vi "Vision Processing.vi"(4 "error in (no error)":errorcluster, 6 "CameraDevRef":T1) -> ()   [LabVIEW 2011]
uses:
  <vilib>/Rock Robotics/WPI/Camera/WPI_CameraDevRef.ctl
  Robot Global Data.vi
  <vilib>/vision/NI_Vision_Development_Module.lvlib
panel:
  in  "Run Calculations":bool
  in  "Manual Overide":bool
  out "Turret Rotation":dbl
  out "Target X Coord":dbl
  out "Target Distance":dbl
  out "Target Y Coord":dbl
  out "Distance Array":dbl[](array[numeric])
  in  "Scaler":dbl=0.85
  in  "Lower Speed Limit":dbl=0.05
  out "Number of Rectangles Visible":dbl
  out "Y Position Array":dbl[](array[numeric])
  out "X Position Array":dbl[](array[numeric])
  in  "View":bool
  out "Target Info":T2(array[cluster])
  in  "Area Size Limit":i32=444
  in  "Particle Count Limit":i32=8
  in  "Score Limits":T3={"Rect Coverage"=76.0, "Aspect Ratio"=40.0, "X Edge Strength"=40.0, "Y Edge Strength"=60.0}
  in  "Processing":enum32{"Color", "Intensity", "Intensity Open"}(tab)=enum."Intensity Open"
  in  "Luminance":i32=255
  in  "Saturation":i32=255
  in  "Hue":i32(knob)=65 scale=0.0..255.0
  in  "Margins":cluster{"Hue":i32, "Sat":i32, "Lum":i32}={"Hue"=20, "Sat"=27, "Lum"=30} {"Sat" scale=0.0..40.0; "Lum" scale=0.0..40.0; "Hue" scale=0.0..40.0}
  in  "Range":cluster{"Lower value":sgl, "Upper value":sgl}={"Lower value"=150.0, "Upper value"=255.0} {"Lower value" scale=0.0..255.0; "Upper value" scale=0.0..255.0}
  in  "Range":cluster{"Lower value":sgl, "Upper value":sgl}={"Lower value"=123.804344, "Upper value"=255.0} {"Lower value" scale=0.0..255.0; "Upper value" scale=0.0..255.0}
  in  "View":bool
  out "Processed Image":T4(plugin-control)
  out "Original Image":T4(plugin-control)
  # "Instructions:\nProcessing the reflective tape that is illuminated by a ring light can be based\non color or light intensity.\nParticles within the image are scored by rectangle coverage, aspect ratio, and\nfor being hollow with a bold edge. A particle is considered a target if all scores\nare above the score limits. Particles can be annotated -- surrounded by\na rectangle and scores drawn to the left .\nTo control the number of particles being scored, use the count limit and the size\nlimit."
  # "To debug, Enable using the View button.\nFor color processing, you can click in the image to select the color for processing."
  # "Enable by clicking the View button.\nGreen scores are above the limit, orange are below. Inner/outer rect\nindicates all passed."
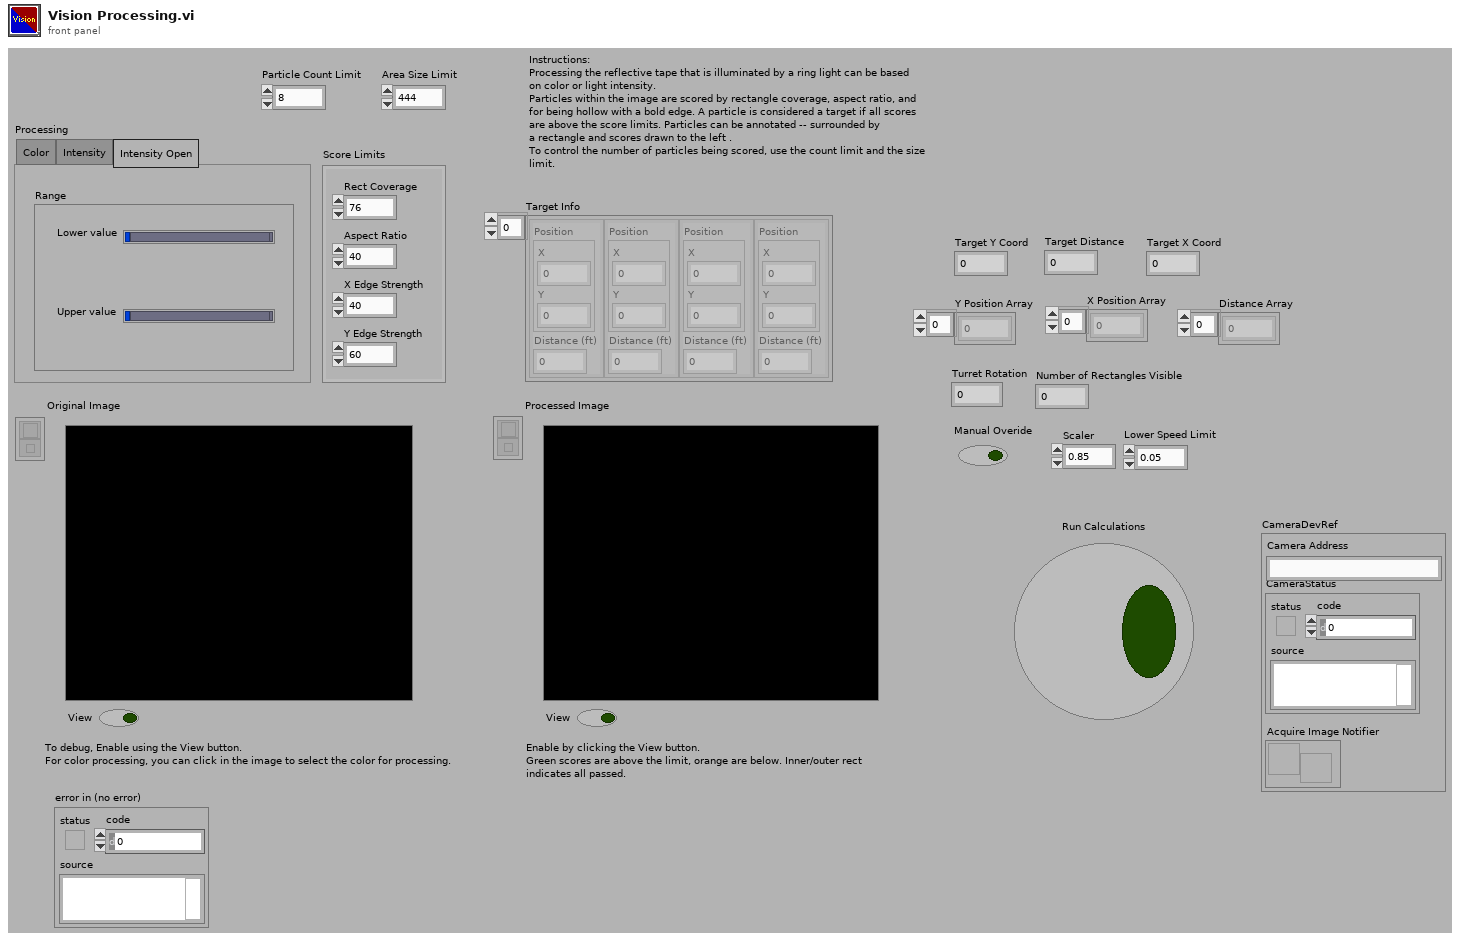
[diagram p1: front panel]
types:
  T1 = typedef "WPI_CameraDevRef.ctl" = cluster{"Camera Address":string, "CameraStatus":errorcluster, "Acquire Image Notifier":refnum<notifier>}
  T2 = cluster{"Position":cluster{"X":dbl, "Y":dbl}, "Distance (ft)":dbl}[]
  T3 = cluster{"Rect Coverage":dbl, "Aspect Ratio":dbl, "X Edge Strength":dbl, "Y Edge Strength":dbl}
  T4 = typedef "IMAQ Image.ctl" = refnum<image>
  T5 = typedef "Image Type" = u32
  T6 = enum32{"AutoM", "Close", "Dilate", "Erode", "Gradient", "Gradient out", "Gradient in", "Hit miss", "Open", "PClose", "POpen", "Thick", "Thin"}
  T7 = typedef "WPI_CameraImageSize.ctl" = enum16{"640x480", "320x240", "160x120"}
  T8 = cluster{"fps":i32, "compression":i32, "Image Size":T7}
  T9 = cluster{cluster{"Left":dbl, "Top":dbl, "Right":dbl, "Bottom":dbl}, dbl[]}[]
  T10 = cluster{"Left":dbl, "Top":dbl, "Right":dbl, "Bottom":dbl}
  T11 = cluster{"Target Center (-1 to 1)":cluster{"X":dbl, "Y":dbl}, "Distance (ft)":dbl}
  T12 = cluster{"Target Center (-1 to 1)":cluster{"X":dbl, "Y":dbl}, "Distance (ft)":dbl}[]
  T13 = cluster{"Axis 1":dbl, "Axis 2":dbl, "Axis 3":dbl, "Axis 4":dbl, "Axis 5":dbl, "Axis 6":dbl, "Button 1":bool, "Button 2":bool, "Button 3":bool, "Button 4":bool, "Button 5":bool, "Button 6":bool, "Button 7":bool, "Button 8":bool, "Button 9":bool, "Button 10":bool, "Button 11":bool, "Button 12":bool}
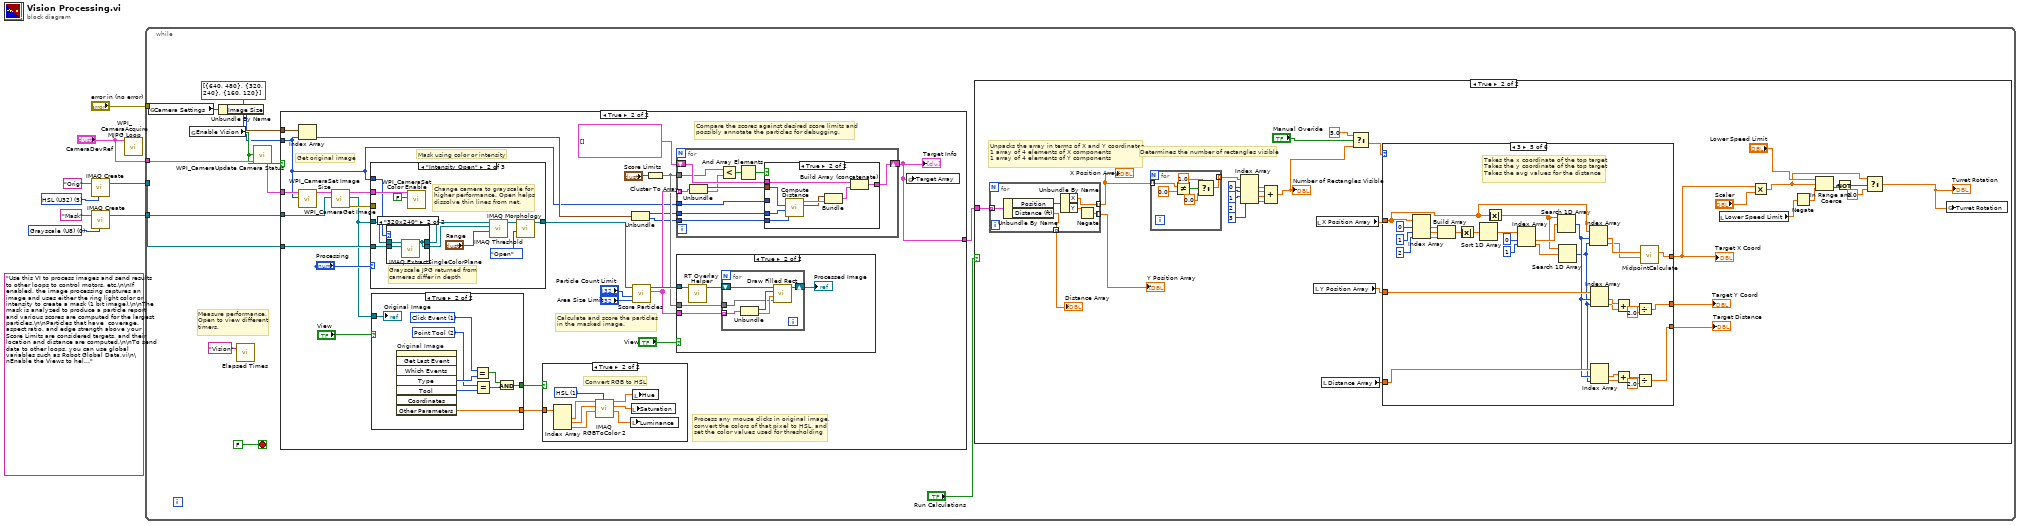
[diagram p0: block diagram]
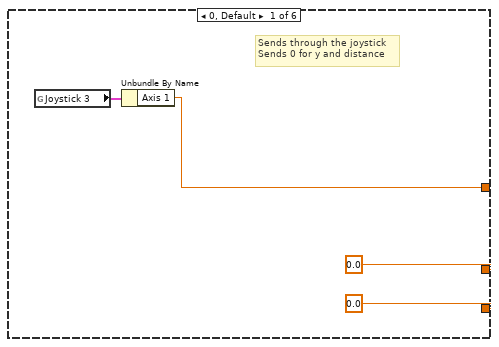
[diagram p3: hidden frame]
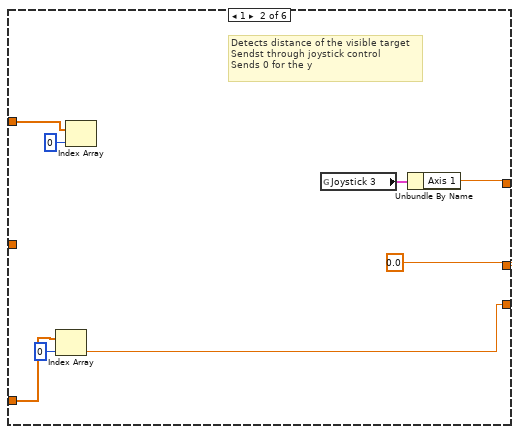
[diagram p4: hidden frame]
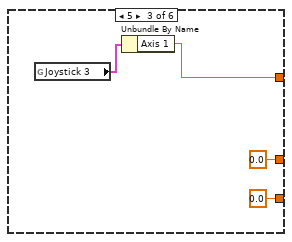
[diagram p5: hidden frame]
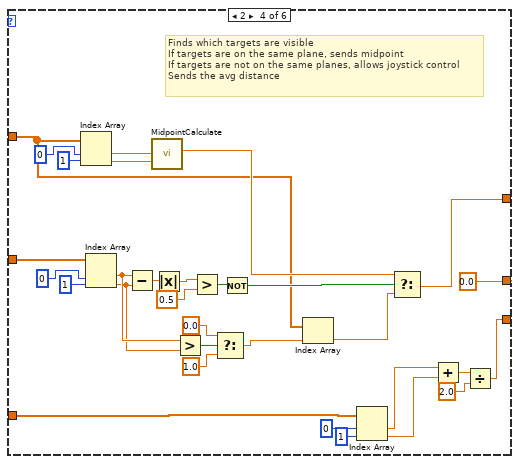
[diagram p6: hidden frame]
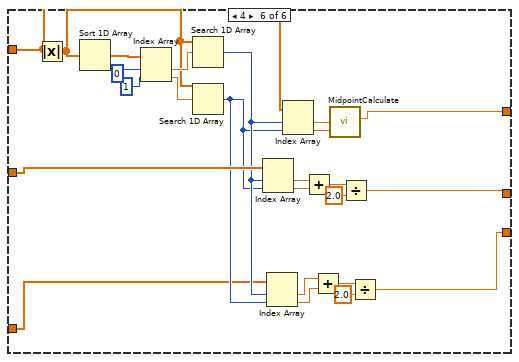
[diagram p7: hidden frame]
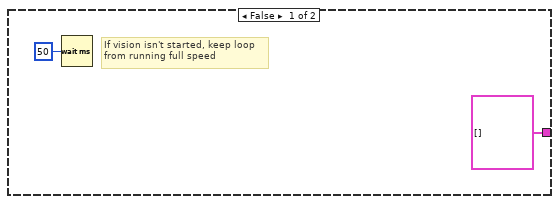
[diagram p8: hidden frame]
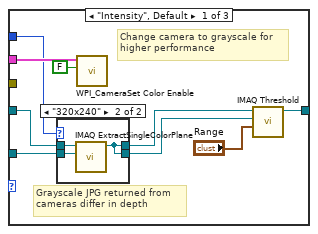
[diagram p10: hidden frame]
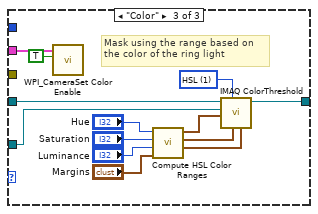
[diagram p13: hidden frame]
diagram:
  w3 = T5 0 items=["Grayscale (U8)", "Grayscale (I16)", "Grayscale (SGL)", "Complex (CSG)", "RGB (U32)", "HSL (U32)", "RGB (U64)", "Grayscale (U16)"] ("Image Type")
  (unwired) "Use this VI to process images and send results to other loops to control motors, etc.\n\nIf enabled, the image processing captures an image and uses either the ring light color or intensity to create a mask (1 bit image).\n\nThe mask is analyzed to produce a particle report and various scores are computed for the largest particles.\n\nParticles that have  coverage, aspect ratio, and edge strength above your Score Limits are considered targets, and their location and distance are computed.\n\nTo send data to other loops, you can use global variables such as Robot Global Data.vi\n\nEnable the Views to help debug color settings. Disable the View to speed up processing."
  w7 = T5 5 items=["Grayscale (U8)", "Grayscale (I16)", "Grayscale (SGL)", "Complex (CSG)", "RGB (U32)", "HSL (U32)", "RGB (U64)", "Grayscale (U16)"] ("Image Type")
  n1 = call "IMAQ Create"("Image Name"="Orig", "Image Type"=w7) -> ("New Image"=w6:T4)  [unwired: 2 in, 2 out]
  n2 = call "IMAQ Create"("Image Name"="Mask", "Image Type"=w3) -> ("New Image"=w1:T4)  [unwired: 2 in, 2 out]
  n3 = call <vilib>:"WPI_CameraAcquire MJPG Loop.vi"("CameraDevRef"="CameraDevRef") -> ()  [unwired: 11 in]
  n4 = while {
    tunnel: w6 -> [w19]
    tunnel: "CameraDevRef" -> [w18]
    tunnel: "error in (no error)" -> [_]
    tunnel: w1 -> [w14]
    stop <- FALSE stop-if-true
    # "Measure performance.\nOpen to view different\ntimers."
    n5 = global read "Robot Global Data.vi" "Camera Settings"() -> (w12:T8)
    n6 = global read "Robot Global Data.vi" "Enable Vision"() -> (w16:bool)
    n7 = Unbundle By Name(w12) -> ("Image Size"=w11:T7)
    n8 = call "Elapsed Times.vi"("Call Name"="Vision") -> ()  [unwired: 2 in, 1 out]
    n9 = call <vilib>:"WPI_CameraUpdate Camera Status.vi"("CameraDevRef In"=w18, "Enable Vision"=w16) -> ("CameraDevRef Out"=w17:T1)  [unwired: 3 in]
    n10 = case shown="True" w16 {
      tunnel: w19 -> [_ w186]
      tunnel: w17 -> [_ w182]
      tunnel: w14 -> [_ w173]
      tunnel: cluster{i32, i32}[] [{640, 480}, {320, 240}, {160, 120}] -> [_ w177]
      tunnel: w11 -> [_ w170]
      tunnel: [T2 [] w171] -> w10
      frame False {
        # "If vision isn't started, keep loop\nfrom running full speed"
        n11 = Wait (ms)(milliseconds to wait=u32 50) -> ()  [unwired: 1 out]
      }
      frame True {
        # "Compare the scores against desired score limits and\npossibly annotate the particles for debugging."
        # "Process any mouse clicks in original image,\nconvert the colors of that pixel to HSL, and\nset the color values used for thresholding"
        # "Calculate and score the particles\nin the masked image."
        # "Mask using color or intensity"
        # "Get original image"
        n12 = call <vilib>:"WPI_CameraSet Image Size.vi"("Image Size"=w170, "CameraDevRef"=w182) -> ("CameraDevRef Out"=w183:T1)  [unwired: 8 in, 1 out]
        n13 = Index Array(array=w177, index=w170) -> (element=w174:cluster{i32, i32})
        n14 = call <vilib>:"WPI_CameraGet Image.vi"("Image"=w186, "CameraDevRef"=w183) -> ("error out"=w184:errorcluster, "Image Out"=w172:T4, "CameraDevRef Out"=w185:T1)  [unwired: 7 in]
        n15 = case shown="\"Intensity Open\"" "Processing" {
          tunnel: w172 -> [w208 w220 w246]
          tunnel: [w211 w225 w245] -> w180
          tunnel: w185 -> [w209 w223 w236]
          tunnel: w184 -> [_ _ _]
          tunnel: w173 -> [w207 w221 w234]
          tunnel: w170 -> [w206 w222 _]
          frame "Intensity", Default {
            # "Grayscale JPG returned from\ncameras differ in depth"
            # "Change camera to grayscale for\nhigher performance"
            n16 = case shown="\"320x240\"" w206 {
              tunnel: w208 -> [w214 w217]
              tunnel: w207 -> [w213 w216]
              tunnel: [w214 w215] -> w205
              tunnel: [w213 w215] -> w204
              frame "640x480", Default {
              }
              frame "320x240" {
                n17 = call "IMAQ ExtractSingleColorPlane"("Image Dst"=w216, "Image Src"=w217) -> ("Image Dst Out"=w215:T4)  [unwired: 8 in, 1 out]
              }
            }
            n18 = call <vilib>:"WPI_CameraSet Color Enable.vi"("Color Enabled"=FALSE, "CameraDevRef"=w209) -> ()  [unwired: 8 in, 2 out]
            n19 = call "IMAQ Threshold"("Range"="Range", "Image Dst"=w204, "Image Src"=w205) -> ("Image Dst Out"=w211:T4)  [unwired: 3 in, 5 out]
          }
          frame "Intensity Open" {
            # "Grayscale JPG returned from\ncameras differ in depth"
            # "Change camera to grayscale for\nhigher performance. Open helps\ndissolve thin lines from net."
            n20 = case shown="\"320x240\"" w222 {
              tunnel: w220 -> [w230 w233]
              tunnel: w221 -> [w229 w232]
              tunnel: [w230 w231] -> w219
              tunnel: [w229 w231] -> w218
              frame "640x480", Default {
              }
              frame "320x240" {
                n21 = call "IMAQ ExtractSingleColorPlane"("Image Dst"=w232, "Image Src"=w233) -> ("Image Dst Out"=w231:T4)  [unwired: 8 in, 1 out]
              }
            }
            n22 = call <vilib>:"WPI_CameraSet Color Enable.vi"("Color Enabled"=FALSE, "CameraDevRef"=w223) -> ()  [unwired: 8 in, 2 out]
            n23 = call "IMAQ Threshold"("Range"="Range", "Image Dst"=w218, "Image Src"=w219) -> ("Image Dst Out"=w226:T4)  [unwired: 3 in, 5 out]
            n24 = call "IMAQ Morphology"("Operation"=T6."Open", "Image Src"=w226) -> ("Image Dst Out"=w225:T4)  [unwired: 8 in, 1 out]
          }
          frame "Color" {
            w244 = u16 1 items=["RGB", "HSL", "HSV", "HSI"] ("Color Mode")
            # "Mask using the range based on\nthe color of the ring light"
            n25 = call <vilib>:"WPI_CameraSet Color Enable.vi"("Color Enabled"=TRUE, "CameraDevRef"=w236) -> ()  [unwired: 8 in, 2 out]
            n26 = call "Compute HSL Color Ranges.vi"("Margins"="Margins", "Luminance"="Luminance", "Saturation"="Saturation", "Hue"="Hue") -> ("Lum Range"=w241:cluster{i32, i32}, "Sat Range"=w242:cluster{i32, i32}, "Hue Range"=w243:cluster{i32, i32})  [unwired: 5 in]
            n27 = call "IMAQ ColorThreshold"("Blue or Luma or Val or Inten Range"=w241, "Green or Sat Range"=w242, "Color Mode"=w244, "Red or Hue Range"=w243, "Image Dst"=w234, "Image Src"=w246) -> ("Image Dst Out"=w245:T4)  [unwired: 4 in, 1 out]
          }
        }
        n28 = case shown="True" "View" {
          tunnel: w172 -> [_ w266]
          tunnel: [_ w261] -> w179
          tunnel: [_ w258] -> w178
          frame False {
          }
          frame True {
            w259 = 2 items=["None", "Selection Tool", "Point Tool", "Line Tool", "Rectangle Tool", "Oval Tool", "Polygon Tool", "ClosedFreehandTool", "Annulus Tool", "Rotated Rectangle Tool", "Zoom Tool", "Pan Tool", "Polyline Tool", "Freehand Tool"] ("Tool")
            w260 = 1 items=["No Event"=0, "Click Event"=1, "Draw Event"=2, "Size Event"=4, "Scroll Event"=5, "Double Click Event"=8] ("Type")
            n29 = invoke on="Original Image" class="ImageControl" method="Get Last Event"() -> ("Type"=w262:i32, "Tool"=w265:i32, "Other Parameters"=w258:sgl[])  [unwired: 8 in, 5 out]
            n30 = Equal?(x=w260, y=w262) -> (x = y?=w263:bool)
            n31 = Equal?(x=w259, y=w265) -> (x = y?=w264:bool)
            n32 = And(x=w263, y=w264) -> (x .and. y?=w261:bool)
            "Original Image" <- w266
          }
        }
        n33 = case shown="True" w179 {
          tunnel: w178 -> [_ w203]
          frame False {
          }
          frame True {
            w202 = u16 1 items=["RGB", "HSL", "HSV", "HSI", "CIE L*a*b*", "CIE XYZ"] ("Color Mode")
            # "Convert RGB to HSL"
            n34 = Index Array(array=w203) -> (element #1=w201:sgl, element #2=w199:sgl, element #3=w197:sgl)  [unwired: 3 in]
            n35 = call "IMAQ RGBToColor 2"("Color Mode"=w202, "Blue value"=w197, "Green value"=w199, "Red value"=w201) -> ("Blue or Luma or Val or Inten or Z or b*value"=w196:dbl, "Green or Sat or Y or a* value"=w198:dbl, "Red or Hue or X or L* value"=w200:dbl)  [unwired: 4 in, 1 out]
            n36 = local write "Luminance"(w196) -> ()
            n37 = local write "Saturation"(w198) -> ()
            n38 = local write "Hue"(w200) -> ()
          }
        }
        n39 = Unbundle(w174) -> (w176:i32, w175:i32)
        n40 = call "Score Particles.vi"("Area Size Limit"="Area Size Limit", "Particle Count Limit"="Particle Count Limit", "Image Refnum in"=w180) -> ("Scored Particle Info"=w191:T9, "Image Refnum out"=w194:T4)  [unwired: 7 in]
        n41 = Cluster To Array(cluster="Score Limits") -> (array=w189:dbl[])
        n42 = for {
          shift-right: [w276] -> w171
          shift-left: T2 [] -> [w277]
          tunnel: w176 -> [w275]
          tunnel: w191 -> [w273] mode=indexing
          tunnel: w189 -> [w268]
          tunnel: w170 -> [w272]
          tunnel: w175 -> [w267]
          n43 = Unbundle(w273) -> (w274:T10, w269:dbl[])
          n44 = Less?(x=w268, y=w269) -> (x < y?=w271:bool[])
          n45 = And Array Elements(Boolean array=w271) -> (logical AND=w270:bool)
          n46 = case shown="True" w270 {
            tunnel: w277 -> [w278 w286]
            tunnel: [w278 w285] -> w276
            tunnel: w274 -> [_ w281]
            tunnel: w275 -> [_ w283]
            tunnel: w272 -> [_ _]
            tunnel: w267 -> [_ w280]
            frame False {
            }
            frame True {
              n47 = call "Compute Distance.vi"("Y Image Resolution"=w280, "X Image Resolution"=w283, "Bounding Box"=w281) -> ("Target Center (-1 to 1)"=w279:cluster{"X":dbl, "Y":dbl}, "Distance (ft)"=w282:dbl)  [unwired: 7 in]
              n48 = Bundle("Target Center (-1 to 1)"=w279, "Distance (ft)"=w282) -> (w284:T11)  [unwired: 1 in]
              n49 = Build Array (concatenate)(w286, w284) -> (w285:T12)
            }
          }
        }
        "Target Info" <- w171
        n50 = case shown="True" "View" {
          tunnel: w194 -> [_ w248]
          tunnel: w191 -> [_ w250]
          tunnel: w189 -> [_ w249]
          frame False {
          }
          frame True {
            n51 = call "RT Overlay Helper.vi"("Refnum in"=w248) -> ("Refnum out"=w251:T4)  [unwired: 10 in]
            n52 = for {
              shift-right: [w256] -> w247
              shift-left: w251 -> [w257]
              tunnel: w250 -> [w253] mode=indexing
              tunnel: w249 -> [w252]
              n53 = Unbundle(w253) -> (w254:T10, w255:dbl[])
              n54 = call "Draw Filled Rect.vi"("Limits"=w252, "Scores"=w255, "Bounding Box"=w254, "image in"=w257) -> ("image out"=w256:T4)  [unwired: 7 in]
            }
            "Processed Image" <- w247
          }
        }
        n55 = global write "Robot Global Data.vi" "Target Array"(w171) -> ()
      }
    }
    n56 = case shown="True" "Run Calculations" {
      tunnel: w10 -> [_ w22]
      frame False {
      }
      frame True {
        # "Determines the number of rectangles visible"
        # "Unpacks the array in terms of X and Y coordinates\n1 array of 4 elements of X components\n1 array of 4 elements of Y components"
        n57 = for {
          tunnel: [w165] -> w23 mode=indexing
          tunnel: [w166] -> w33 mode=indexing
          tunnel: w22 -> [w163] mode=indexing
          tunnel: [w162] -> w42 mode=indexing
          n58 = Unbundle By Name(w163) -> ("Position"=w167:cluster{"X":dbl, "Y":dbl}, "Distance (ft)"=w162:dbl)
          n59 = Unbundle By Name(w167) -> ("X"=w166:dbl, "Y"=w164:dbl)
          n60 = Negate(x=w164) -> (-x=w165:dbl)
        }
        "X Position Array" <- w33
        "Y Position Array" <- w23
        "Distance Array" <- w42
        n61 = for {
          tunnel: w33 -> [w57] mode=indexing
          tunnel: [w53] -> w32 mode=indexing
          n62 = Not Equal?(x=w57, y=0.0) -> (x != y?=w56:bool)
          n63 = Select(t=1.0, s=w56, f=0.0) -> (s? t:f=w53:dbl)
        }
        n64 = Index Array(array=w32, index #1=0 ("index"), index #2=1 ("index"), index #3=2 ("index"), index #4=3 ("index")) -> (element #1=w30:dbl, element #2=w31:dbl, element #3=w29:dbl, element #4=w28:dbl)
        n65 = Compound Arithmetic op=ADD(w30, w31, w29, w28) -> (w21:dbl)
        "Number of Rectangles Visible" <- w21
        n66 = local read "Y Position Array"() -> (w46:dbl[])
        n67 = local read "X Position Array"() -> (w34:dbl[])
        n68 = local read "Distance Array"() -> (w47:dbl[])
        n69 = Select(t=5.0, s="Manual Overide", f=w21) -> (s? t:f=w50:dbl)
        n70 = case shown="3" w50 {
          tunnel: w34 -> [_ w65 _ w76 w123 w156]
          tunnel: [w61 w63 w73 w94 w120 w153] -> w45
          tunnel: [0.0 ("X") 0.0 ("X") 0.0 ("X") 0.0 ("X") w111 w147] -> w43
          tunnel: [0.0 ("X") w68 0.0 ("X") w87 w106 w139] -> w44
          tunnel: w46 -> [_ _ _ w103 w119 w152]
          tunnel: w47 -> [_ w70 _ w86 w118 w144]
          frame 0, Default {
            # "Sends through the joystick\nSends 0 for y and distance"
            n71 = global read "Robot Global Data.vi" "Joystick 3"() -> (w62:T13)
            n72 = Unbundle By Name(w62) -> ("Axis 1"=w61:dbl)
          }
          frame 1 {
            # "Detects distance of the visible target\nSendst through joystick control\nSends 0 for the y"
            n73 = Index Array(array=w70, index=0) -> (element=w68:dbl)
            n74 = Index Array(array=w65, index=0) -> ()  [unwired: 1 out]
            n75 = global read "Robot Global Data.vi" "Joystick 3"() -> (w64:T13)
            n76 = Unbundle By Name(w64) -> ("Axis 1"=w63:dbl)
          }
          frame 5 {
            n77 = global read "Robot Global Data.vi" "Joystick 3"() -> (w74:T13)
            n78 = Unbundle By Name(w74) -> ("Axis 1"=w73:dbl)
          }
          frame 2 {
            # "Finds which targets are visible\nIf targets are on the same plane, sends midpoint\nIf targets are not on the same planes, allows joystick control\nSends the avg distance"
            n79 = Index Array(array=w76, index #1=0 ("index"), index #2=1 ("index")) -> (element #1=w92:dbl, element #2=w91:dbl)
            n80 = Index Array(array=w103, index #1=0 ("index"), index #2=1 ("index")) -> (element #1=w82:dbl, element #2=w81:dbl)
            n81 = Subtract(x=w82, y=w81) -> (x-y=w100:dbl)
            n82 = call "MidpointCalculate.vi"("X2"=w91, "X1"=w92) -> ("Midpoint"=w95:dbl)  [unwired: 9 in]
            n83 = Absolute Value(x=w100) -> (abs(x)=w99:dbl)
            n84 = Greater?(x=w82, y=w81) -> (0:w80:bool)
            n85 = Greater?(x=w99, y=0.5) -> (0:w96:bool)
            n86 = Select(t=0.0, s=w80, f=1.0) -> (s? t:f=w77:dbl)
            n87 = Not(x=w96) -> (.not. x?=w97:bool)
            n88 = Index Array(array=w76, index=w77) -> (element=w75:dbl)
            n89 = Index Array(array=w86, index #1=0 ("index"), index #2=1 ("index")) -> (element #1=w85:dbl, element #2=w84:dbl)
            n90 = Select(t=w95, s=w97, f=w75) -> (s? t:f=w94:dbl)
            n91 = Add(x=w85, y=w84) -> (x+y=w90:dbl)
            n92 = Divide(x=w90, y=2.0) -> (x/y=w87:dbl)
          }
          frame 3 {
            # "Takes the x coordinate of the top target\nTakes the y coordinate of the top target\nTakes the avg values for the distance"
            n93 = Index Array(array=w123, index #1=0 ("index"), index #2=1 ("index"), index #3=2 ("index")) -> (element #1=w134:dbl, element #2=w133:dbl, element #3=w132:dbl)
            n94 = Build Array(w134, w133, w132) -> (w131:dbl[])
            n95 = Absolute Value(x=w131) -> (abs(x)=w130:dbl[])
            n96 = Sort 1D Array(array=w130) -> (sorted array=w129:dbl[])
            n97 = Absolute Value(x=w123) -> (abs(x)=w124:dbl[])
            n98 = Index Array(array=w129, index #1=0 ("index"), index #2=1 ("index")) -> (element #1=w126:dbl, element #2=w125:dbl)
            n99 = Search 1D Array(1D array=w124, element=w126) -> (index of element=w117:i32)  [unwired: 1 in]
            n100 = Search 1D Array(1D array=w124, element=w125) -> (index of element=w116:i32)  [unwired: 1 in]
            n101 = Index Array(array=w123, index #1=w117, index #2=w116) -> (element #1=w122:dbl, element #2=w121:dbl)
            n102 = Index Array(array=w119, index #1=w117, index #2=w116) -> (element #1=w113:dbl, element #2=w112:dbl)
            n103 = Index Array(array=w118, index #1=w117, index #2=w116) -> (element #1=w108:dbl, element #2=w107:dbl)
            n104 = Add(x=w113, y=w112) -> (x+y=w115:dbl)
            n105 = Add(x=w108, y=w107) -> (x+y=w110:dbl)
            n106 = Divide(x=w115, y=2.0) -> (x/y=w111:dbl)
            n107 = Divide(x=w110, y=2.0) -> (x/y=w106:dbl)
            n108 = call "MidpointCalculate.vi"("X2"=w121, "X1"=w122) -> ("Midpoint"=w120:dbl)  [unwired: 9 in]
          }
          frame 4 {
            n109 = Absolute Value(x=w156) -> (abs(x)=w138:dbl[])
            n110 = Sort 1D Array(array=w138) -> (sorted array=w161:dbl[])
            n111 = Index Array(array=w161, index #1=0 ("index"), index #2=1 ("index")) -> (element #1=w157:dbl, element #2=w158:dbl)
            n112 = Search 1D Array(1D array=w138, element=w157) -> (index of element=w146:i32)  [unwired: 1 in]
            n113 = Search 1D Array(1D array=w138, element=w158) -> (index of element=w145:i32)  [unwired: 1 in]
            n114 = Index Array(array=w152, index #1=w146, index #2=w145) -> (element #1=w150:dbl, element #2=w151:dbl)
            n115 = Index Array(array=w144, index #1=w146, index #2=w145) -> (element #1=w141:dbl, element #2=w140:dbl)
            n116 = Index Array(array=w156, index #1=w146, index #2=w145) -> (element #1=w155:dbl, element #2=w154:dbl)
            n117 = Add(x=w150, y=w151) -> (x+y=w149:dbl)
            n118 = Add(x=w141, y=w140) -> (x+y=w142:dbl)
            n119 = call "MidpointCalculate.vi"("X2"=w154, "X1"=w155) -> ("Midpoint"=w153:dbl)  [unwired: 9 in]
            n120 = Divide(x=w149, y=2.0) -> (x/y=w147:dbl)
            n121 = Divide(x=w142, y=2.0) -> (x/y=w139:dbl)
          }
        }
        "Target Y Coord" <- w43
        "Target Distance" <- w44
        "Target X Coord" <- w45
        n122 = local read "Lower Speed Limit"() -> (w36:dbl)
        n123 = Multiply(x=w45, y="Scaler") -> (x*y=w41:dbl)
        n124 = Negate(x=w36) -> (-x=w37:dbl)
        n125 = In Range and Coerce(upper limit="Lower Speed Limit", x=w41, lower limit=w37) -> (In Range?=w38:bool)  [unwired: 1 out]
        n126 = Not(x=w38) -> (.not. x?=w39:bool)
        n127 = Select(t=w41, s=w39, f=0.0) -> (s? t:f=w52:dbl)
        "Turret Rotation" <- w52
        n128 = global write "Robot Global Data.vi" "Turret Rotation"(w52) -> ()
      }
    }
  }
